vi "Edit Module Name.vi"(7 "Theme":bool, 8 "error in":errorcluster, 11 "Value":variant) -> (0 "error out":errorcluster, 2 "Canceled":bool, 3 "New Module Name":string)   [LabVIEW 2019, in "Panther Dashboard.lvlib"]
uses:
  Panther Dashboard.lvlib
panel:
  in  "Continue":bool
  in  "Cancel":bool
  in  "Module Name":string
  # "A VI named \"Module Name--constant.vi\" acts as an identifier for your DQMH module.\nBy default, its value matches the name of the DQMH library containing the module.\n\nDQMH Framework offers a scripting tool to rename the module. You can access it through:\n   \nTools menu->DQMH Consortium->DQMH -> Module -> Rename DQMH Module\n\nReasons to Change Module Name--constant.vi:\n\nManual Library Rename: If you manually renamed the library and want the \"Module Name--constant.vi\" to reflect this change.\nClarity and Consistency: If you want the \"Module Name--constant.vi\" to be more descriptive and different from the library name. This can improve code readability, especially if the application contains multiple modules."
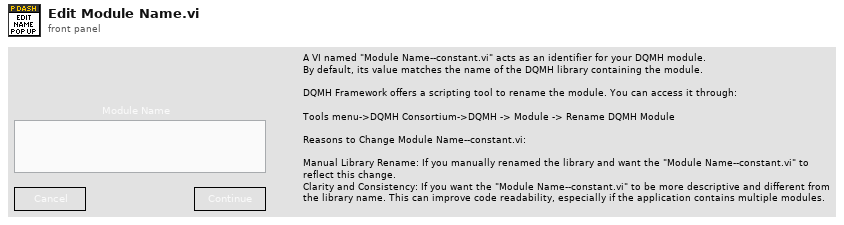
[diagram p1: front panel]
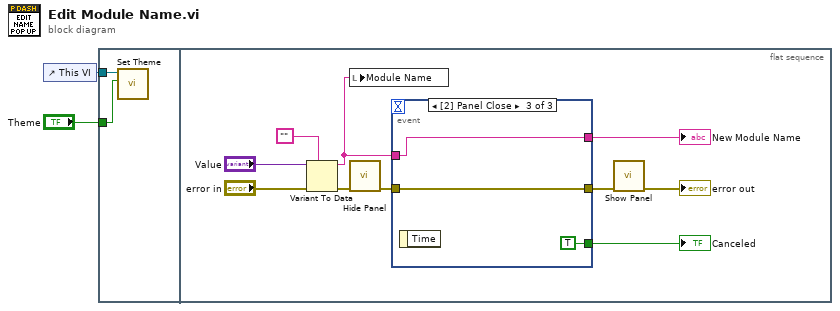
[diagram p0: block diagram]
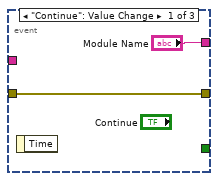
[diagram p2: hidden frame]
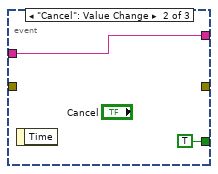
[diagram p3: hidden frame]
diagram:
  n1 = control-ref of="This VI"() -> (w2:refnum<vi>)
  n2 = flat-sequence {
    tunnel: w2 -> [w4]
    tunnel: "Theme" -> [w3]
    frame #0 {
      n3 = call "Set Theme.vi"("Dark?"=w3, "VI in"=w4) -> ()  [unwired: 10 in]
    }
    frame #1 {
      n4 = Variant To Data(error in="error in", type="", Variant="Value") -> (data=w9:string, error out=w12:errorcluster)
      n5 = local write "Module Name"(w9) -> ()
      n6 = call "Hide Panel.vi"("error in (no error)"=w12) -> ("error out"=w13:errorcluster)  [unwired: 10 in]
      n7 = event shown="[2] Panel Close" {
        selector: _ -> [_ _ _]
        dyn-events: _ -> [_ _ _]
        timeout: _ -> [_ _ _]
        tunnel: ["Module Name" w18 w19] -> w8
        tunnel: w9 -> [_ w18 w19]
        tunnel: [w16 _ w21] -> w14
        tunnel: w13 -> [w16 _ w21]
        tunnel: [_ TRUE ("Cancel Button") TRUE ("Cancel Button")] -> w5
        event "Continue": Value Change {
          n8 = event-data() -> ()  [unwired: 1 in, 1 out]
        }
        event "Cancel": Value Change {
          n9 = event-data() -> ()  [unwired: 1 in, 1 out]
        }
        event Panel Close {
          n10 = event-data() -> ()  [unwired: 1 in, 1 out]
        }
      }
      "New Module Name" <- w8
      "Canceled" <- w5
      n11 = call "Show Panel.vi"("error in (no error)"=w14) -> ("error out"=→"error out":errorcluster)  [unwired: 10 in]
    }
  }
